vi "CreatePublicEvents.vi"(8 "error in (no error)":errorcluster, 11 "Subsystem":refnum<class "DAQmx(AI).lvclass">) -> (0 "error out":errorcluster, 3 "Subsystem out":refnum<class "DAQmx(AI).lvclass">)   [LabVIEW 2019, in "DAQmx(AI).lvclass"]
doc: "---------------------------------------------------------------\nJKI State Machine Objects™\nhttp://jki.net/state-machine-objects/\nCopyright (C) 2005-2015, JKI <info@jki.net>\nALL RIGHTS RESERVEDJKI State Machine Objects (SMO) 1.0.0.5\nJKI - JKI\nCopyright (c) 2016, JKI"
uses:
  DAQmx(AI).lvclass
  Typedefs/DataChanged--EventData--Cluster.ctl
  Typedefs/Configuration--Cluster.ctl
  Typedefs/Units -- Enum.ctl
  Typedefs/ScalingEvent--Cluster.ctl
  Typedefs/Scaling(MapRange)--Cluster.ctl
  DAQmx(AI).lvclass/DAQmx(AI).ctl
  vi.lib/JKI/JKI SMO/SMO/SMO.lvclass
panel:
  # "For instructions on how to use the JKI State Machine Objects, examples and video tutorials, visit:\nhttp://jki.net/state-machine-objects/\n\nJKI State Machine Objects™\nhttp://jki.net/state-machine-objects/\nCopyright (C) 2005-2015, JKI <info@jki.net>\nALL RIGHTS RESERVED"
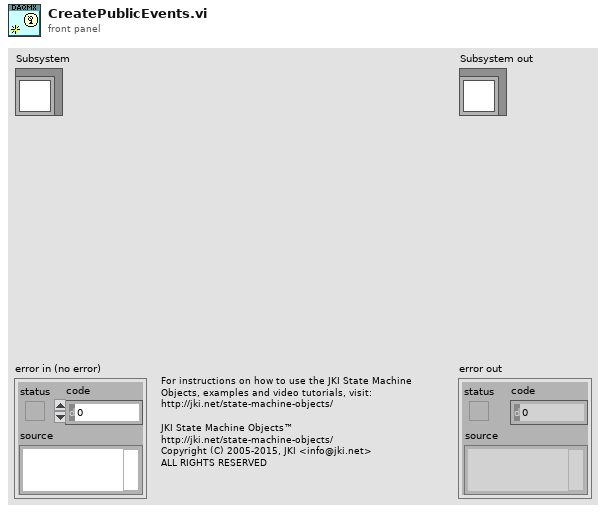
[diagram p1: front panel]
types:
  T1 = typedef "DAQmx(AI).lvclass/ScalingEvent--Cluster.ctl" = cluster{"Scale Name":string, "Units":string, "Range":T2}
  T2 = typedef "DAQmx(AI).lvclass/Scaling(MapRange)--Cluster.ctl" = cluster{"Minimum":dbl, "Maximum":dbl}
  T3 = typedef "DAQmx(AI).lvclass/Configuration--Cluster.ctl" = cluster{"PhysChan":tag, "Period (ms)":i64, "input terminal cfg":i32, "minimum value":dbl, "maximum value":dbl, "units":T4, "task name":string, "TDMS File Path":path, "Group Name":string}
  T4 = typedef "DAQmx(AI).lvclass/Units -- Enum.ctl" = enum16{"Volts", "Amps", "Deg F", "Deg C", "Deg R", "Kelvins", "Strain", "Ohms", "Hz", "Seconds", "Meters", "Inches", "Degrees", "Radians", "Ticks", "g", "m/s^2", "m/s", "in/s", "Pascals", "Newtons", "Pounds", "kgf", "psi", "bar", "Nm", "oz-in", "lb-in", "lb-ft", "Volts/Volt", "mVolts/Volt", "From TEDS"}
  T5 = typedef "DAQmx(AI).lvclass/DataChanged--EventData--Cluster.ctl" = cluster{"Timestamp":timestamp, "Value":dbl}
  T6 = typedef "DAQmx(AI).lvclass/PrivateData--Ref.ctl" = refnum<data-value>
  T7 = typedef "DAQmx(AI).lvclass/PrivateData--Cluster.ctl" = cluster{"Configuration":T3, "Public Events":T8, "Data":dbl, "Scaling":T9, "Private Events":T14}
  T8 = typedef "DAQmx(AI).lvclass/PublicEvents--Cluster.ctl" = cluster{"Value Changed":refnum<user-event>, "Task Configuration":refnum<user-event>, "Scaling":refnum<user-event>}
  T9 = typedef "DAQmx(AI).lvclass/Scaling--Cluster.ctl" = cluster{"Scale Name":string, "Scale Type":T10, "Scaled Units":string, "Linear":T11, "Map Range":T2, "Polynomial":T12, "Table":T13}
  T10 = typedef "DAQmx(AI).lvclass/ScalingType--Enum.ctl" = enum16{"No scaling", "Linear", "Map Range", "Polynomial", "Table"}
  T11 = typedef "DAQmx(AI).lvclass/Scaling(Linear)--Cluster.ctl" = cluster{"Slope":dbl, "Intercept":dbl}
  T12 = typedef "DAQmx(AI).lvclass/Scaling(Polynomial)--Cluster.ctl" = cluster{"forward coeff":dbl[], "reverse coeff":dbl[]}
  T13 = typedef "DAQmx(AI).lvclass/Scaling(Table)--Cluster.ctl" = cluster{"scaled values":dbl[], "pres-scaled values":dbl[]}
  T14 = typedef "DAQmx(AI).lvclass/PrivateEvents--Cluster.ctl" = cluster{"Logging":refnum<user-event>}
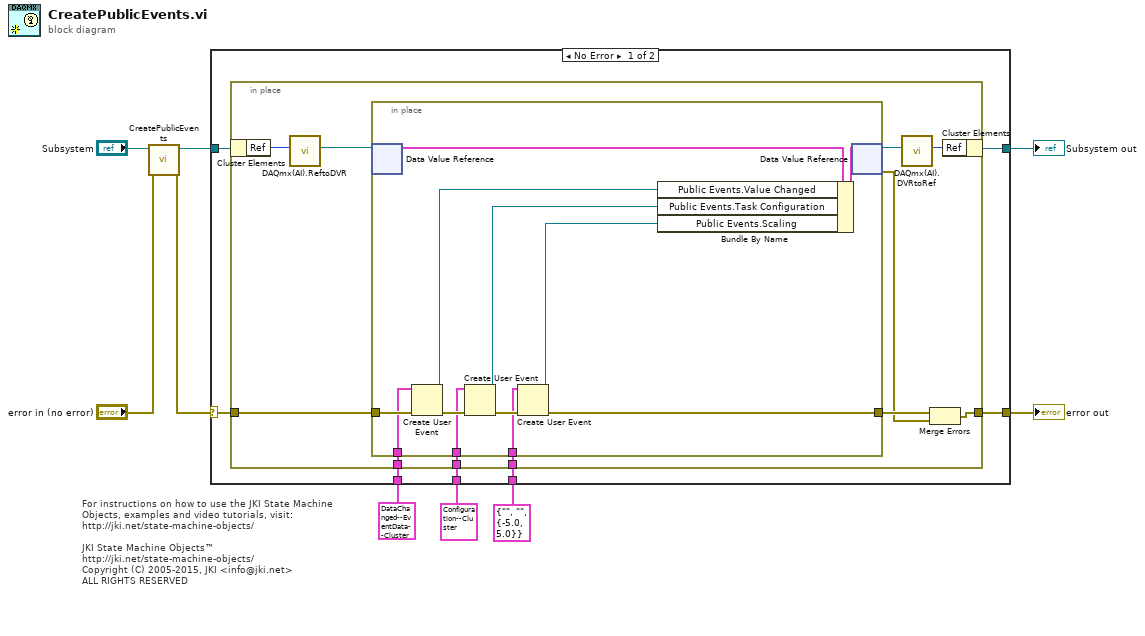
[diagram p0: block diagram]
diagram:
  # "For instructions on how to use the JKI State Machine Objects, examples and video tutorials, visit:\nhttp://jki.net/state-machine-objects/\n\nJKI State Machine Objects™\nhttp://jki.net/state-machine-objects/\nCopyright (C) 2005-2015, JKI <info@jki.net>\nALL RIGHTS RESERVED"
  n1 = call-parent "CreatePublicEvents.vi"("error in (no error)"="error in (no error)", "SMO"="Subsystem") -> ("error out"=w3:errorcluster, "SMO out"=w5:refnum<class "DAQmx(AI).lvclass">)  [unwired: 8 in]
  n2 = case shown="No Error" w3 {
    selector: w3 -> [w14 w41]
    tunnel: [w13 w41] -> w8
    tunnel: [w15 w40] -> w9
    tunnel: w5 -> [w16 w40]
    tunnel: T5 {"Timestamp"=timestamp(0 s since 1904-01-01), "Value"=0.0} ("Data In Event Data") -> [w12 _]
    tunnel: T3 {"PhysChan"="SMO-Sim/ai0", "Period (ms)"=50, "input terminal cfg"=-1, "minimum value"=0.0, "maximum value"=0.0, "units"=enum."Volts", "task name"="", "TDMS File Path"=path "", "Group Name"=""} ("Configuration") -> [w11 _]
    tunnel: T1 {"Scale Name"="", "Units"="", "Range"={"Minimum"=-5.0, "Maximum"=5.0}} ("Scaling Event") -> [w10 _]
    frame No Error {
      n3 = in-place {
        in-place-border: w14 -> [w27]
        in-place-border: [w24] -> w13
        in-place-border: w12 -> [w23]
        in-place-border: w11 -> [w18]
        in-place-border: w10 -> [w17]
        n4 = in-place-cluster #1(w16) -> ("Ref"=w22:u32)
        n5 = call "DAQmx(AI).ReftoDVR.vi"("Ref"=w22) -> ("Ref"=w21:T6)  [unwired: 10 in]
        n6 = in-place {
          in-place-border: w27 -> [w37]
          in-place-border: [w30] -> w26
          in-place-border: w23 -> [w36]
          in-place-border: w18 -> [w33]
          in-place-border: w17 -> [w29]
          n7 = in-place-dvr #2(w21) -> (w38:T7)  [unwired: 1 out]
          n8 = Create User Event(user event datatype=w36, error in=w37) -> (user event=w34:refnum<user-event>, error out=w35:errorcluster)
          n9 = Create User Event(user event datatype=w33, error in=w35) -> (user event=w32:refnum<user-event>, error out=w31:errorcluster)
          n10 = Create User Event(user event datatype=w29, error in=w31) -> (user event=w28:refnum<user-event>, error out=w30:errorcluster)
          n11 = Bundle By Name(cluster=w38, "Public Events.Value Changed"=w34, "Public Events.Task Configuration"=w32, "Public Events.Scaling"=w28) -> (w39:T7)
          n12 = in-place-dvr #2(w39) -> (w20:T6, w25:errorcluster)
        }
        n13 = call "DAQmx(AI).DVRtoRef.vi"("Ref"=w20) -> ("Ref"=w19:u32)  [unwired: 10 in]
        n14 = Merge Errors(w26, w25) -> (w24:errorcluster)
        n15 = in-place-cluster #1("Ref"=w19) -> (w15:refnum<class "DAQmx(AI).lvclass">)
      }
    }
    frame Error {
    }
  }
  "error out" <- w8
  "Subsystem out" <- w9
